vi "1A Interpret NMEA Sentence.vi"(10 "Defilter Wind Data":bool=TRUE, 11 "NMEA Sentence":string) -> ()   [LabVIEW 2011]
doc: "Interprets the NMEA 0813 sentences that we are using from our Airmar PB200 WeatherStation sensor.\nBy Jaime McCandless\nTODO: finish implementing NMEA sentences"
uses:
  2-Think/2 Typedefs/UTM Location.ctl
  2-Think/2 Typedefs/heading.ctl
  2-Think/2 Typedefs/Velocity.ctl
  2-Think/2 Typedefs/apparent wind.ctl
  2-Think/2 Typedefs/pitch and roll.ctl
  2-Think/2 Globals/2 Global.vi
  <vilib>/regexp/Match Regular Expression.xnode
panel:
  out "Meteorological Data":T1
  in  "UTC Time Zone":i32=-5
  in  "Tab Control":T2(tab)
  out "GPS (GGA) Data":T3
  out "GPS (GLL) Data":T4
  out "GPGSA Data":T5
  out "UTC Time":timestamp
  out "Local Time":timestamp
  out "Lattitude (ddmm.mmmm)":dbl format="%_8g"
  out "Lattitude North/South":string
  out "Longitude (ddmm.mmmm)":dbl format="%_8g"
  out "Longitude East/West":string
  out "Speed over ground (knots)":dbl format="%_3g"
  out "Course over ground (degrees)":dbl format="%_4g"
  out "Magnetic Variation (degrees)":dbl format="%_4g"
  out "Variation East/West":string
  out "GPS (RMC) Data":T6 {"Course over ground (degrees)" format="%#.6g"; "Speed over ground (knots)" format="%#.6g"; "Magnetic Variation (degrees)" format="%#.6g"; "Longitude (ddmm.mmmm)" format="%#.6g"; "Lattitude (ddmm.mmmm)" format="%#.6g"}
  out "GPS Data Valid?":bool
  out "Robot UTM Location":T7 {"North" format="%#_10f"; "East" format="%#_8f"}
  out "GPS (VTG) Data":T8
  out "Heading":dbl
  out "Turn (ROT) Data":T9
  out "Wind (MWV) Data":T10
  out "Transducer (XDR) B Data":cluster{"Pitch (deg)":dbl, "Roll (deg)":dbl}
  out "Transducer (XDR) A Data":T11
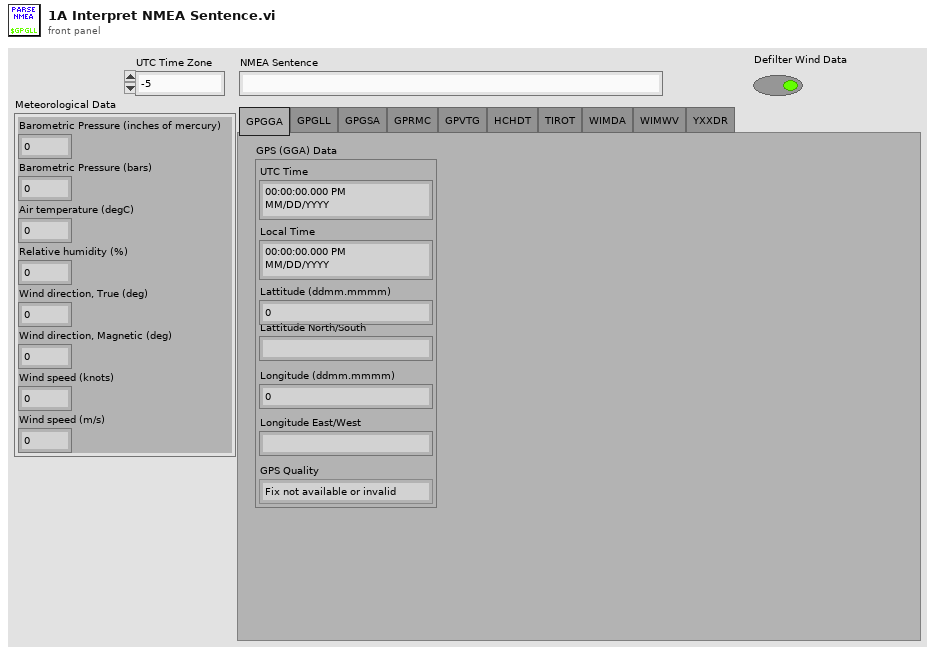
[diagram p1: front panel]
types:
  T1 = cluster{"Barometric Pressure (inches of mercury)":dbl, "Barometric Pressure (bars)":dbl, "Air temperature (degC)":dbl, "Relative humidity (%)":dbl, "Wind direction, True (deg)":dbl, "Wind direction, Magnetic (deg)":dbl, "Wind speed (knots)":dbl, "Wind speed (m/s)":dbl}
  T2 = enum32{"GPGGA", "GPGLL", "GPGSA", "GPRMC", "GPVTG", "HCHDT", "TIROT", "WIMDA", "WIMWV", "YXXDR"}
  T3 = cluster{"UTC Time":timestamp, "Local Time":timestamp, "Lattitude (ddmm.mmmm)":dbl, "Lattitude North/South":string, "Longitude (ddmm.mmmm)":dbl, "Longitude East/West":string, "GPS Quality":enum16{"Fix not available or invalid", "GPS SPS Mode, fix valid", "Differential GPS, SPS Mode, fix valid", "GPS PPS Mode, fix valid", "Real Time Kinematic (RTK)", "Float RTK", "Estimated (dead reckoning) Mode", "Manual Input Mode", "Simulator Mode"}}
  T4 = cluster{"UTC Time":timestamp, "Local Time":timestamp, "Lattitude (ddmm.mmmm)":dbl, "Lattitude North/South":string, "Longitude (ddmm.mmmm)":dbl, "Longitude East/West":string, "GPS Mode":string, "GPS Data Valid?":bool}
  T5 = cluster{"Mode":string, "Fix Strength":i32, "Satellite IDs":i32[], "PDOP":dbl, "HDOP":dbl, "VDOP":dbl}
  T6 = cluster{"UTC Time":timestamp, "Local Time":timestamp, "Lattitude (ddmm.mmmm)":dbl, "Lattitude North/South":string, "Longitude (ddmm.mmmm)":dbl, "Longitude East/West":string, "Magnetic Variation (degrees)":dbl, "Variation East/West":string, "Speed over ground (knots)":dbl, "Course over ground (degrees)":dbl}
  T7 = typedef "UTM Location.ctl" = cluster{"UTM Zone":dbl, "Hemisphere":enum16{"North", "South"}, "East":dbl, "North":dbl}
  T8 = cluster{"Course Over Ground (True)":dbl, "Course Over Ground (Magnetic)":dbl, "Speed Over Ground (Knots)":dbl, "Speed Over Ground (km/hr)":dbl, "GPS Mode":string}
  T9 = cluster{"Rate of Turn (deg/min)":dbl, "Turn Rotation Data Valid?":bool}
  T10 = cluster{"Angle relative to boat (deg)":dbl, "Wind Data Valid?":bool, "Wind speed (knots)":dbl, "True (T) or Relative (R)":string}
  T11 = cluster{"Calc. Relative Wind Chill (degC)":dbl, "Calc. Theoretical Wind Chill (degC)":dbl, "Calc. Heat Index (degC)":dbl, "Meas. Barometric Pressure (bars)":dbl}
  T12 = cluster{"second":i32, "minute":i32, "hour":i32, "day of month":i32, "month":i32, "year":i32, "day of week":i32, "day of year":i32, "is DST":i32}
  T13 = typedef "heading.ctl" = dbl
  T14 = typedef "Velocity.ctl" = cluster{"East":dbl, "North":dbl}
  T15 = typedef "apparent wind.ctl" = cluster{"Toward Fore":dbl, "Toward Starboard":dbl}
  T16 = typedef "pitch and roll.ctl" = cluster{"Pitch":dbl, "Roll":dbl}
  T17 = typedef "generalized sensor status.ctl" = cluster{"Sensor Connected":T18, "Sensor Initialized":T18, "Sensor OK":T18, "Latest Error String":string, "GPS Lock":T18}
  T18 = typedef "indicator LED.ctl" = bool
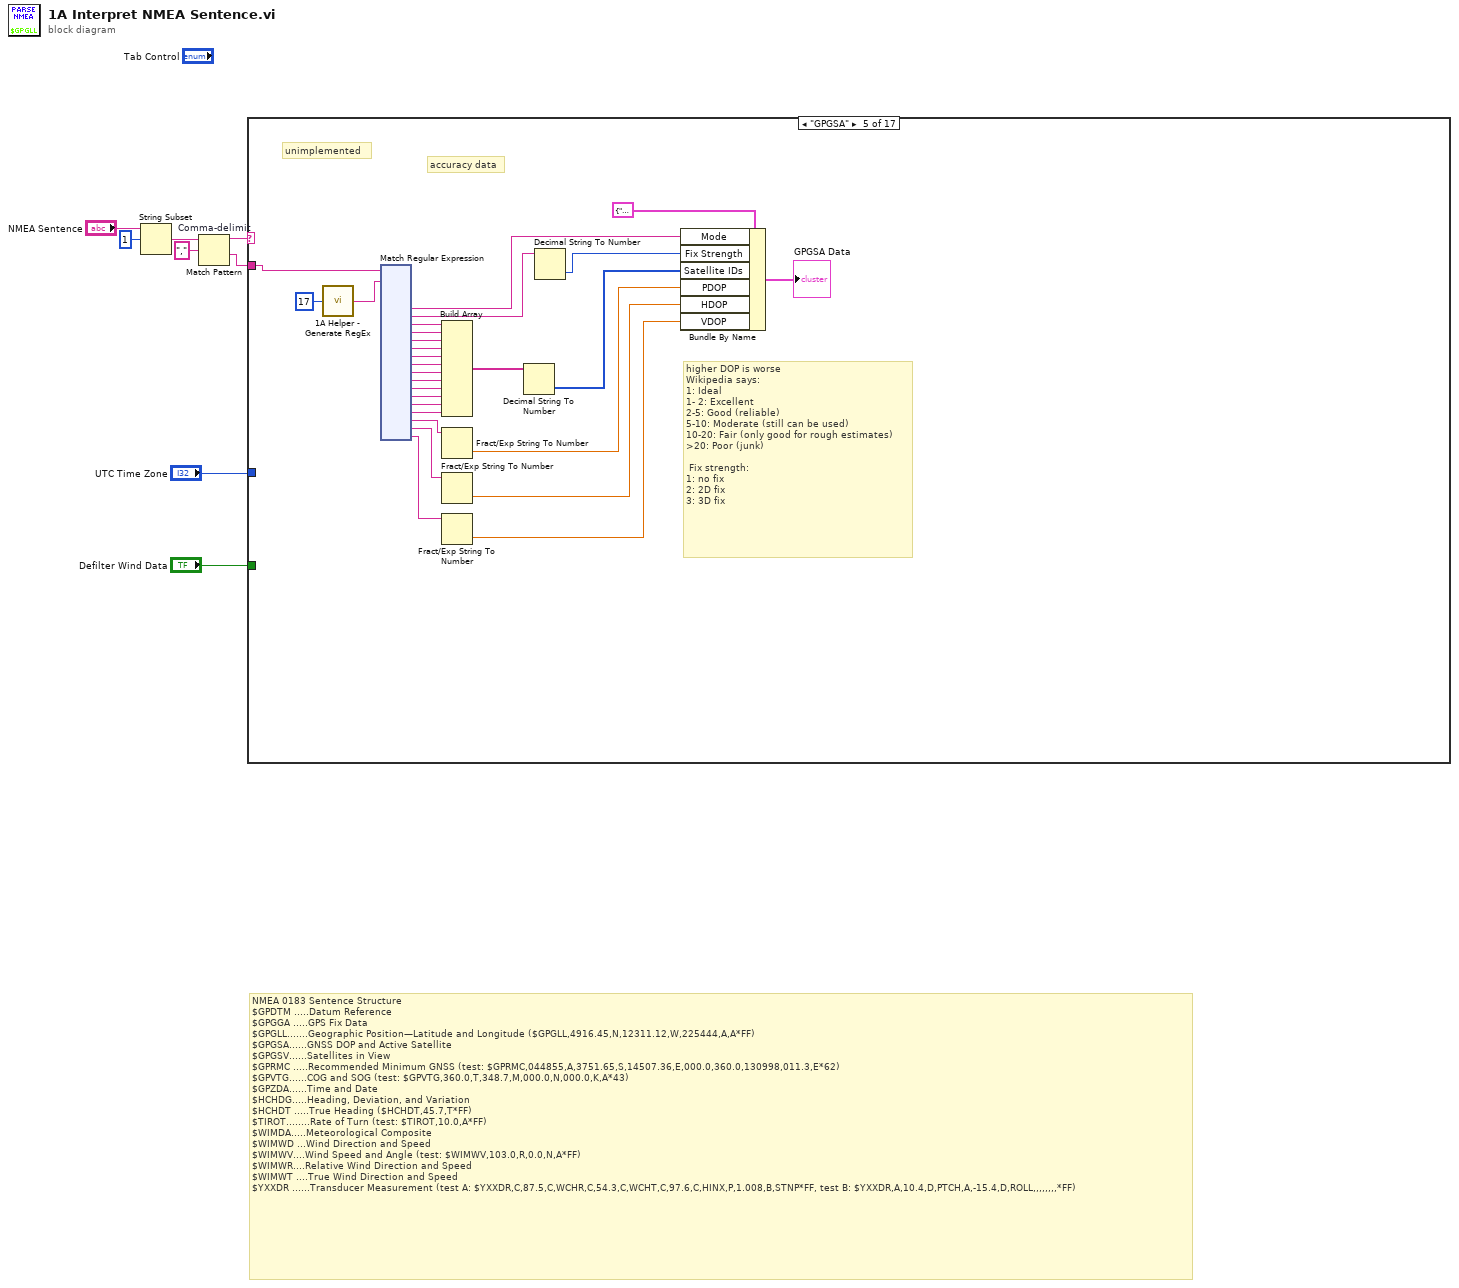
[diagram p0: block diagram]
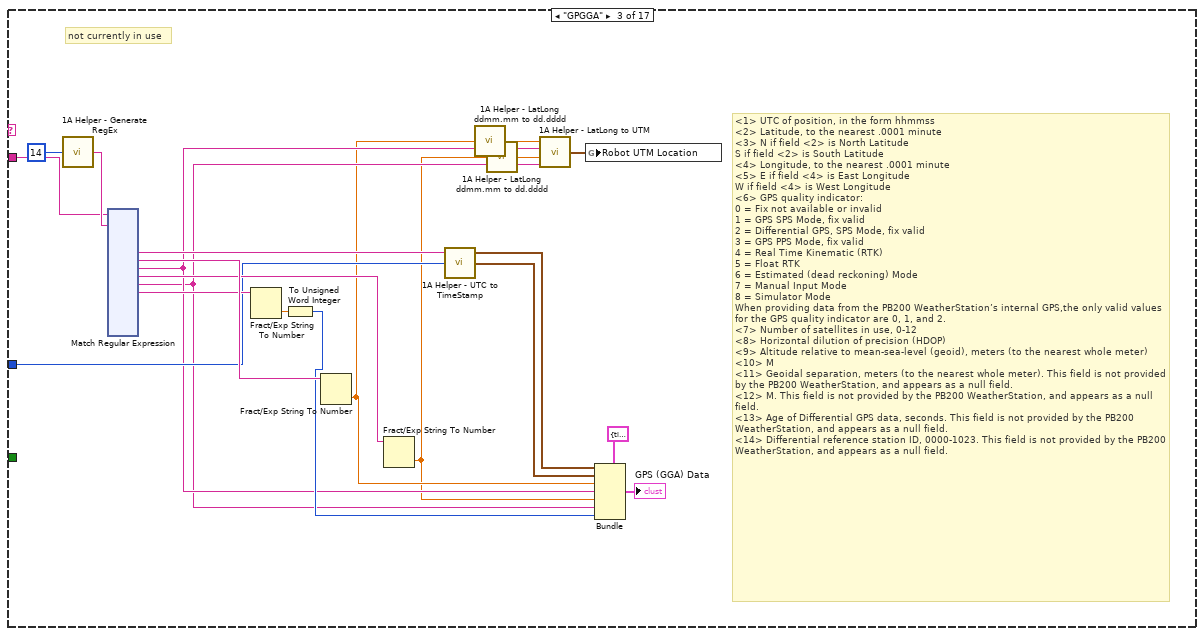
[diagram p4: hidden frame]
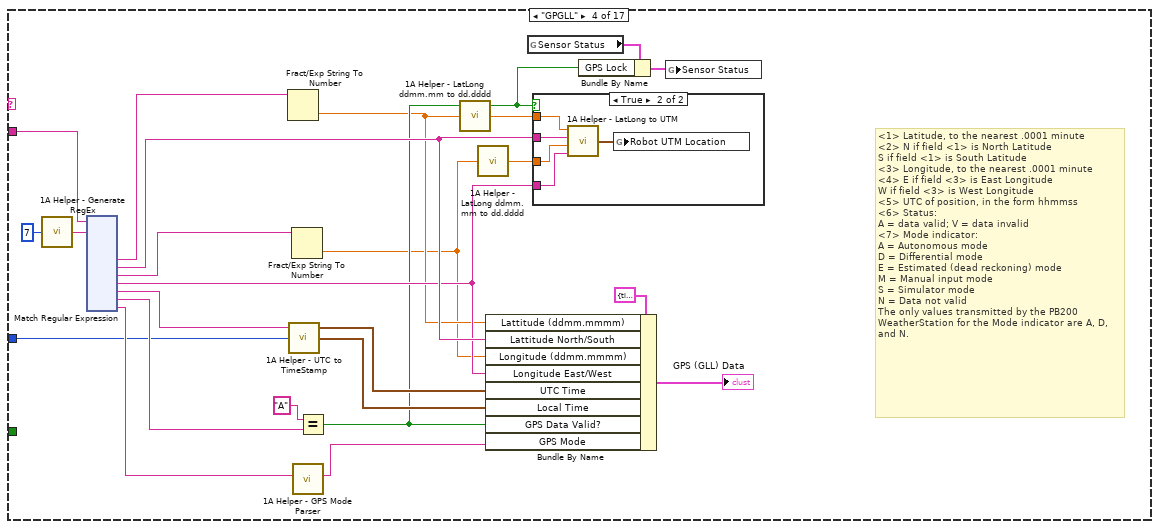
[diagram p5: hidden frame]
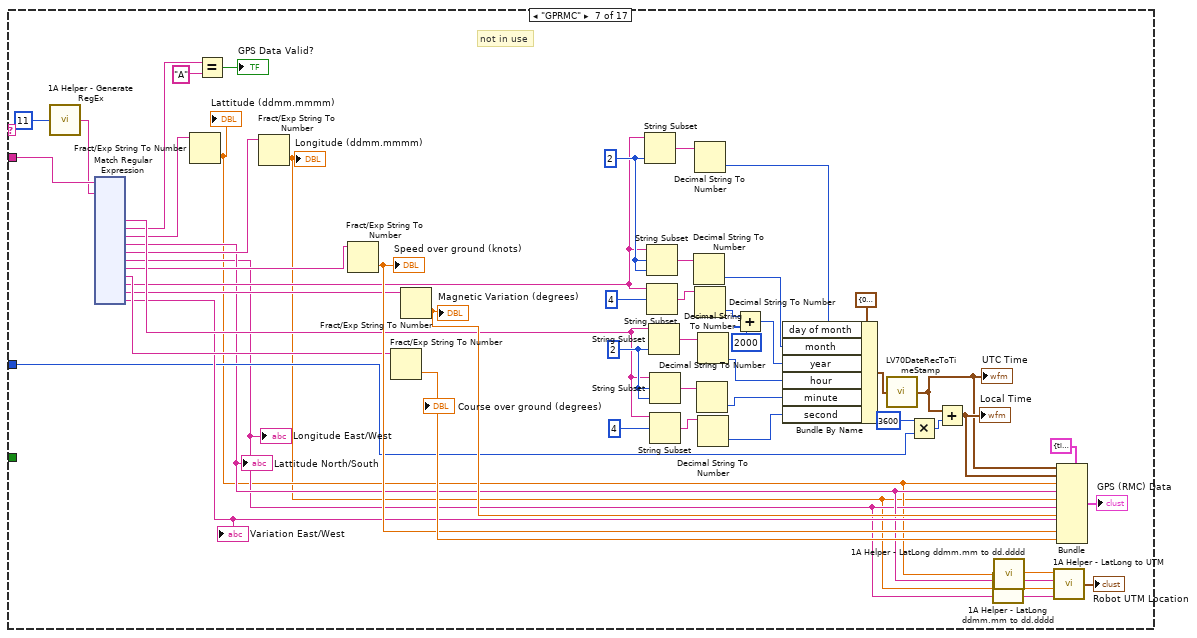
[diagram p8: hidden frame]
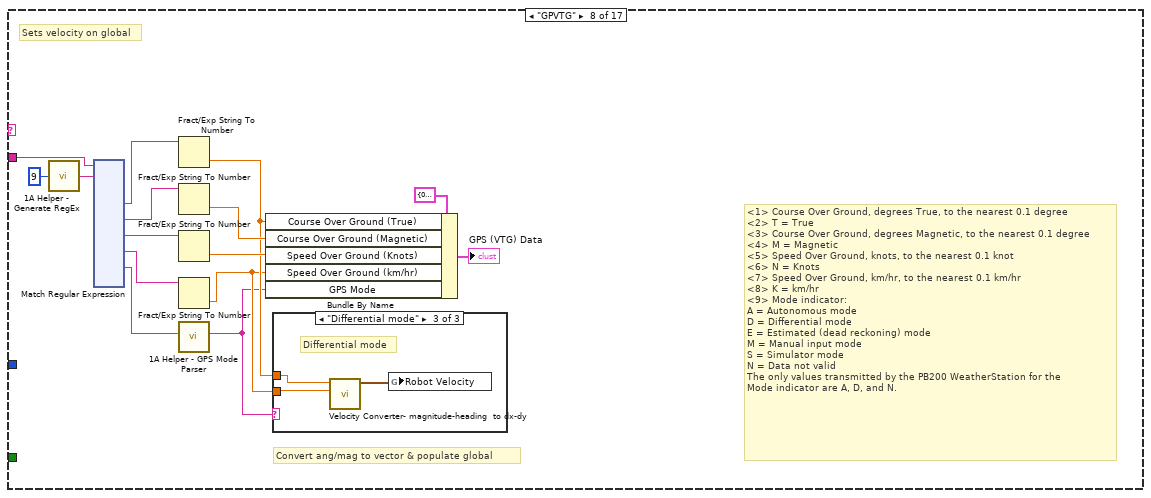
[diagram p9: hidden frame]
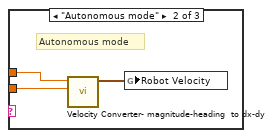
[diagram p11: hidden frame]
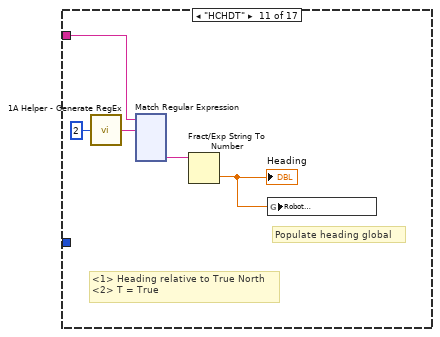
[diagram p14: hidden frame]
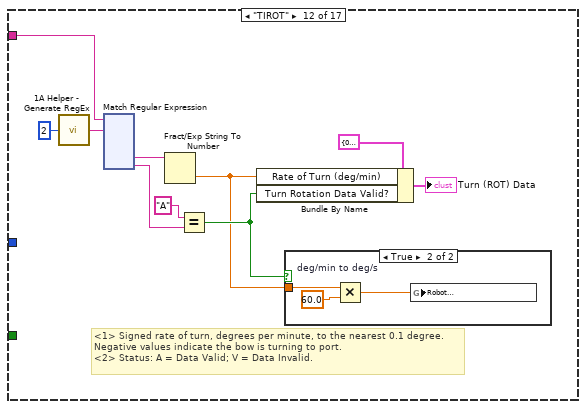
[diagram p15: hidden frame]
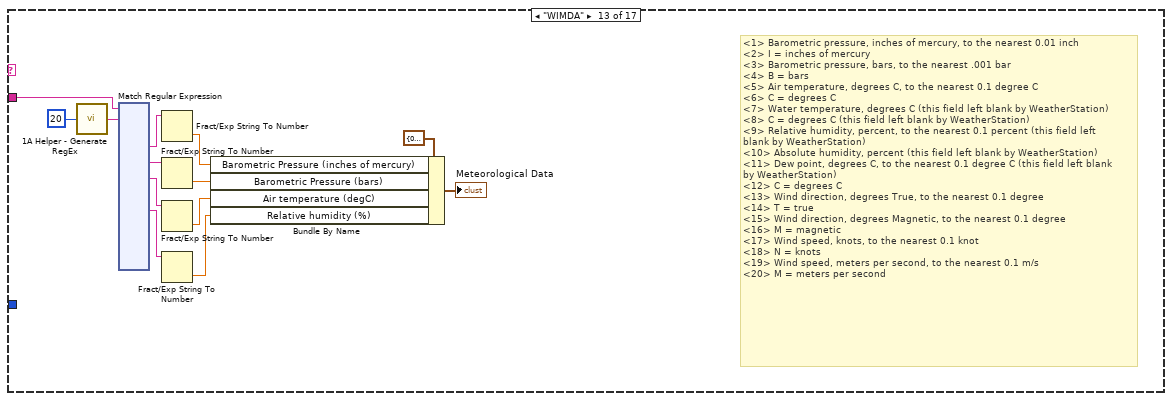
[diagram p17: hidden frame]
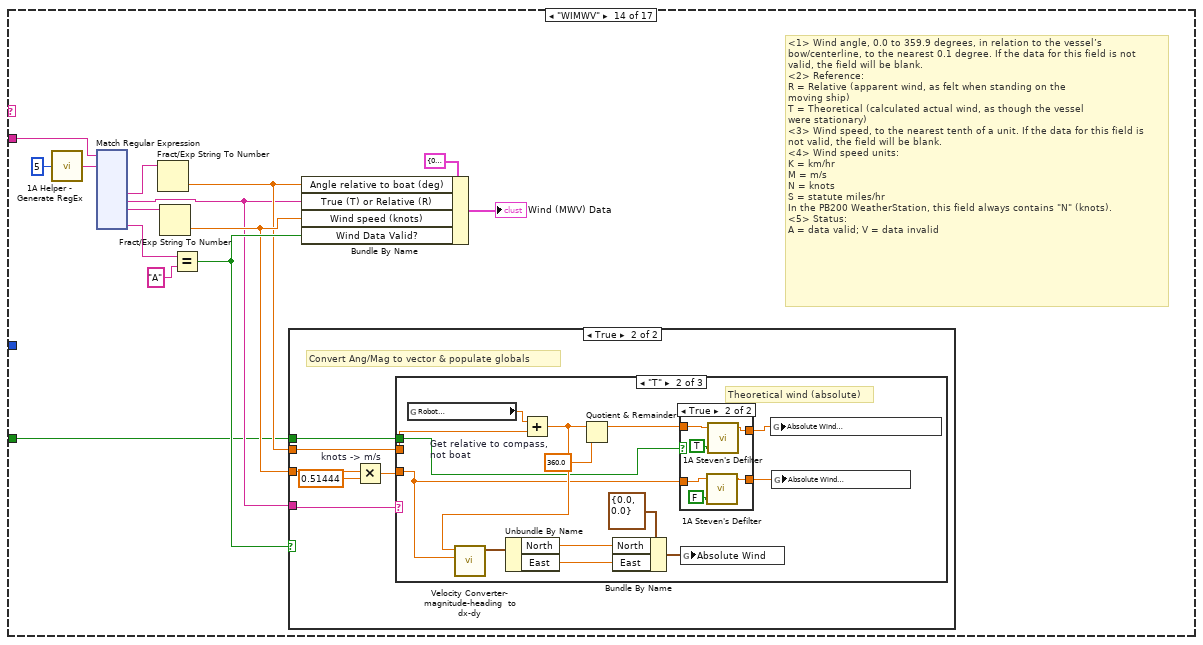
[diagram p18: hidden frame]
diagram:
  # "NMEA 0183 Sentence Structure\n$GPDTM .....Datum Reference\n$GPGGA .....GPS Fix Data\n$GPGLL.......Geographic Position—Latitude and Longitude ($GPGLL,4916.45,N,12311.12,W,225444,A,A*FF)\n$GPGSA......GNSS DOP and Active Satellite\n$GPGSV......Satellites in View\n$GPRMC .....Recommended Minimum GNSS (test: $GPRMC,044855,A,3751.65,S,14507.36,E,000.0,360.0,130998,011.3,E*62)\n$GPVTG......COG and SOG (test: $GPVTG,360.0,T,348.7,M,000.0,N,000.0,K,A*43)\n$GPZDA......Time and Date\n$HCHDG.....Heading, Deviation, and Variation\n$HCHDT .....True Heading ($HCHDT,45.7,T*FF)\n$TIROT........Rate of Turn (test: $TIROT,10.0,A*FF)\n$WIMDA.....Meteorological Composite\n$WIMWD ...Wind Direction and Speed\n$WIMWV....Wind Speed and Angle (test: $WIMWV,103.0,R,0.0,N,A*FF)\n$WIMWR....Relative Wind Direction and Speed\n$WIMWT ....True Wind Direction and Speed\n$YXXDR ......Transducer Measurement (test A: $YXXDR,C,87.5,C,WCHR,C,54.3,C,WCHT,C,97.6,C,HINX,P,1.008,B,STNP*FF, test B: $YXXDR,A,10.4,D,PTCH,A,-15.4,D,ROLL,,,,,,,,*FF)"
  n1 = String Subset(string="NMEA Sentence", offset (0)=1) -> (substring=w5:string)  [unwired: 1 in]
  n2 = Match Pattern "Comma-delimit"(string=w5, regular expression=",") -> (before substring=w6:string, after substring=w7:string)  [unwired: 1 in, 2 out]
  n3 = case shown="\"GPGSA\"" w6 {
    tunnel: w7 -> [_ _ w27 w171 w328 _ w477 w644 _ _ w778 w900 w1031 w1171 _ _ w1339]
    tunnel: "UTC Time Zone" -> [_ _ w16 w163 _ _ w465 _ _ _ _ _ _ _ _ _ _]
    tunnel: "Defilter Wind Data" -> [_ _ _ _ _ _ _ _ _ _ _ _ _ w1162 _ _ _]
    frame "", Default {
    }
    frame "GPDTM" {
      # "unimplemented"
    }
    frame "GPGGA" {
      # "not currently in use"
      # "<1> UTC of position, in the form hhmmss\n<2> Latitude, to the nearest .0001 minute\n<3> N if field <2> is North Latitude\nS if field <2> is South Latitude\n<4> Longitude, to the nearest .0001 minute\n<5> E if field <4> is East Longitude\nW if field <4> is West Longitude\n<6> GPS quality indicator:\n0 = Fix not available or invalid\n1 = GPS SPS Mode, fix valid\n2 = Differential GPS, SPS Mode, fix valid\n3 = GPS PPS Mode, fix valid\n4 = Real Time Kinematic (RTK)\n5 = Float RTK\n6 = Estimated (dead reckoning) Mode\n7 = Manual Input Mode\n8 = Simulator Mode\nWhen providing data from the PB200 WeatherStation’s internal GPS,the only valid values for the GPS quality indicator are 0, 1, and 2.\n<7> Number of satellites in use, 0-12\n<8> Horizontal dilution of precision (HDOP)\n<9> Altitude relative to mean-sea-level (geoid), meters (to the nearest whole meter)\n<10> M\n<11> Geoidal separation, meters (to the nearest whole meter). This field is not provided by the PB200 WeatherStation, and appears as a null field.\n<12> M. This field is not provided by the PB200 WeatherStation, and appears as a null field.\n<13> Age of Differential GPS data, seconds. This field is not provided by the PB200 WeatherStation, and appears as a null field.\n<14> Differential reference station ID, 0000-1023. This field is not provided by the PB200 WeatherStation, and appears as a null field."
      n4 = call "1A Helper - Generate RegEx.vi"("# Datums"=14) -> ("RegEx"=w28:string)
      n5 = xnode "Match Regular Expression"("input string"=w27, "regular expression"=w28) -> ("submatch 1"=w19:string, "submatch 2"=w25:string, "submatch 3"=w14:string, "submatch 4"=w24:string, "submatch 5"=w13:string, "submatch 6"=w23:string)  [unwired: 4 in, 10 out]
      n6 = Fract/Exp String To Number(string=w23) -> (number=w22:dbl)  [unwired: 3 in, 1 out]
      n7 = To Unsigned Word Integer(number=w22) -> (unsigned 16bit integer=w21:u16)
      n8 = Fract/Exp String To Number(string=w25) -> (number=w11:dbl)  [unwired: 3 in, 1 out]
      n9 = Fract/Exp String To Number(string=w24) -> (number=w9:dbl)  [unwired: 3 in, 1 out]
      n10 = call "1A Helper - UTC to TimeStamp.vi"("UTC Time Zone in"=w16, "UTC (hhmmss)"=w19) -> ("Local Time"=w17:timestamp, "UTC Time"=w18:timestamp)  [unwired: 2 in]
      n11 = call "1A Helper - LatLong ddmm.mm to dd.dddd.vi"("Lattitude/Longitude in ddmm.mmmm"=w11) -> ("Latitude/Longitude in dd.dddddd"=w12:dbl)
      n12 = call "1A Helper - LatLong ddmm.mm to dd.dddd.vi"("Lattitude/Longitude in ddmm.mmmm"=w9) -> ("Latitude/Longitude in dd.dddddd"=w10:dbl)
      n13 = call "1A Helper - LatLong to UTM.vi"("East/West"=w13, "Longitude"=w10, "North/South"=w14, "Latitude"=w12) -> ("Robot UTM Location"=w15:T7)
      n14 = global write "2 Global.vi" "Robot UTM Location"(w15) -> ()
      n15 = Bundle(cluster=T3 {"UTC Time"=timestamp(0 s since 1904-01-01), "Local Time"=timestamp(0 s since 1904-01-01), "Lattitude (ddmm.mmmm)"=0.0, "Lattitude North/South"="", "Longitude (ddmm.mmmm)"=0.0, "Longitude East/West"="", "GPS Quality"=enum."GPS SPS Mode, fix valid"} ("Cluster"), "UTC Time"=w18, "Local Time"=w17, "Lattitude (ddmm.mmmm)"=w11, "Lattitude North/South"=w14, "Longitude (ddmm.mmmm)"=w9, "Longitude East/West"=w13, "GPS Quality"=w21) -> (→"GPS (GGA) Data":T3)
    }
    frame "GPGLL" {
      # "<1> Latitude, to the nearest .0001 minute\n<2> N if field <1> is North Latitude\nS if field <1> is South Latitude\n<3> Longitude, to the nearest .0001 minute\n<4> E if field <3> is East Longitude\nW if field <3> is West Longitude\n<5> UTC of position, in the form hhmmss\n<6> Status:\nA = data valid; V = data invalid\n<7> Mode indicator:\nA = Autonomous mode\nD = Differential mode\nE = Estimated (dead reckoning) mode\nM = Manual input mode\nS = Simulator mode\nN = Data not valid\nThe only values transmitted by the PB200 WeatherStation for the Mode indicator are A, D, and N."
      n16 = call "1A Helper - Generate RegEx.vi"("# Datums"=7) -> ("RegEx"=w175:string)
      n17 = xnode "Match Regular Expression"("input string"=w171, "regular expression"=w175) -> ("submatch 1"=w174:string, "submatch 2"=w161:string, "submatch 3"=w173:string, "submatch 4"=w160:string, "submatch 5"=w170:string, "submatch 6"=w166:string, "submatch 7"=w172:string)  [unwired: 4 in, 5 out]
      n18 = Fract/Exp String To Number(string=w174) -> (number=w156:dbl)  [unwired: 3 in, 1 out]
      n19 = call "1A Helper - UTC to TimeStamp.vi"("UTC Time Zone in"=w163, "UTC (hhmmss)"=w170) -> ("Local Time"=w165:timestamp, "UTC Time"=w164:timestamp)  [unwired: 2 in]
      n20 = Fract/Exp String To Number(string=w173) -> (number=w154:dbl)  [unwired: 3 in, 1 out]
      n21 = call "1A Helper - GPS Mode Parser.vi"("GPS Mode (Char)"=w172) -> ("GPS Mode (Description)"=w168:string)  [unwired: 6 in]
      n22 = Equal?(x="A" ("y"), y=w166) -> (x = y?=w157:bool)
      n23 = call "1A Helper - LatLong ddmm.mm to dd.dddd.vi"("Lattitude/Longitude in ddmm.mmmm"=w156) -> ("Latitude/Longitude in dd.dddddd"=w155:dbl)
      n24 = call "1A Helper - LatLong ddmm.mm to dd.dddd.vi"("Lattitude/Longitude in ddmm.mmmm"=w154) -> ("Latitude/Longitude in dd.dddddd"=w153:dbl)
      n25 = Bundle By Name(cluster=T4 {"UTC Time"=timestamp(0 s since 1904-01-01), "Local Time"=timestamp(0 s since 1904-01-01), "Lattitude (ddmm.mmmm)"=0.0, "Lattitude North/South"="", "Longitude (ddmm.mmmm)"=0.0, "Longitude East/West"="", "GPS Mode"="", "GPS Data Valid?"=FALSE} ("Cluster"), "Lattitude (ddmm.mmmm)"=w156, "Lattitude North/South"=w161, "Longitude (ddmm.mmmm)"=w154, "Longitude East/West"=w160, "UTC Time"=w164, "Local Time"=w165, "GPS Data Valid?"=w157, "GPS Mode"=w168) -> (→"GPS (GLL) Data":T4)
      n26 = global read "2 Global.vi" "Sensor Status"() -> (w158:T17)
      n27 = case shown="True" w157 {
        tunnel: w155 -> [_ w181]
        tunnel: w161 -> [_ w180]
        tunnel: w153 -> [_ w179]
        tunnel: w160 -> [_ w178]
        frame False {
        }
        frame True {
          n28 = call "1A Helper - LatLong to UTM.vi"("East/West"=w178, "Longitude"=w179, "North/South"=w180, "Latitude"=w181) -> ("Robot UTM Location"=w177:T7)
          n29 = global write "2 Global.vi" "Robot UTM Location"(w177) -> ()
        }
      }
      n30 = Bundle By Name(cluster=w158, "GPS Lock"=w157) -> (w159:T17)
      n31 = global write "2 Global.vi" "Sensor Status"(w159) -> ()
    }
    frame "GPGSA" {
      # "higher DOP is worse\nWikipedia says:\n1: Ideal\n1- 2: Excellent\n2-5: Good (reliable)\n5-10: Moderate (still can be used)\n10-20: Fair (only good for rough estimates)\n>20: Poor (junk)\n\n Fix strength: \n1: no fix\n2: 2D fix\n3: 3D fix"
      # "accuracy data"
      # "unimplemented"
      n32 = call "1A Helper - Generate RegEx.vi"("# Datums"=17) -> ("RegEx"=w327:string)
      n33 = xnode "Match Regular Expression"("input string"=w328, "regular expression"=w327) -> ("submatch 1"=w324:string, "submatch 2"=w323:string, "submatch 3"=w321:string, "submatch 4"=w320:string, "submatch 5"=w319:string, "submatch 6"=w318:string, "submatch 7"=w317:string, "submatch 8"=w316:string, "submatch 9"=w315:string, "submatch 10"=w314:string, "submatch 11"=w313:string, "submatch 12"=w312:string, "submatch 13"=w311:string, "submatch 14"=w310:string, "submatch 15"=w307:string, "submatch 16"=w305:string, "submatch 17"=w303:string)  [unwired: 4 in, 5 out]
      n34 = Build Array(w321, w320, w319, w318, w317, w316, w315, w314, w313, w312, w311, w310) -> (w309:string[])
      n35 = Fract/Exp String To Number(string=w307) -> (number=w306:dbl)  [unwired: 3 in, 1 out]
      n36 = Fract/Exp String To Number(string=w305) -> (number=w304:dbl)  [unwired: 3 in, 1 out]
      n37 = Fract/Exp String To Number(string=w303) -> (number=w302:dbl)  [unwired: 3 in, 1 out]
      n38 = Decimal String To Number(string=w309) -> (number=w308:i32[])  [unwired: 2 in, 1 out]
      n39 = Decimal String To Number(string=w323) -> (number=w322:i32)  [unwired: 2 in, 1 out]
      n40 = Bundle By Name(cluster=T5 {"Mode"="", "Fix Strength"=0, "Satellite IDs"=[], "PDOP"=0.0, "HDOP"=0.0, "VDOP"=0.0} ("GPGSA Data"), "Mode"=w324, "Fix Strength"=w322, "Satellite IDs"=w308, "PDOP"=w306, "HDOP"=w304, "VDOP"=w302) -> (→"GPGSA Data":T5)
    }
    frame "GPGSV" {
      # "unimplemented"
    }
    frame "GPRMC" {
      w495 = 2 ("length (rest)")
      w485 = 2 ("length (rest)")
      # "not in use"
      n41 = call "1A Helper - Generate RegEx.vi"("# Datums"=11) -> ("RegEx"=w467:string)
      n42 = xnode "Match Regular Expression"("input string"=w477, "regular expression"=w467) -> ("submatch 1"=w476:string, "submatch 2"=w475:string, "submatch 3"=w474:string, "submatch 4"=w464:string, "submatch 5"=w473:string, "submatch 6"=w463:string, "submatch 7"=w472:string, "submatch 8"=w471:string, "submatch 9"=w470:string, "submatch 10"=w469:string, "submatch 11"=w468:string)  [unwired: 4 in, 5 out]
      "Lattitude North/South" <- w464
      "Longitude East/West" <- w463
      "Variation East/West" <- w468
      n43 = Fract/Exp String To Number(string=w474) -> (number=w460:dbl)  [unwired: 3 in, 1 out]
      "Lattitude (ddmm.mmmm)" <- w460
      n44 = Equal?(x=w475, y="A") -> (x = y?=→"GPS Data Valid?":bool)
      n45 = Fract/Exp String To Number(string=w473) -> (number=w458:dbl)  [unwired: 3 in, 1 out]
      "Longitude (ddmm.mmmm)" <- w458
      n46 = Fract/Exp String To Number(string=w472) -> (number=w505:dbl)  [unwired: 3 in, 1 out]
      "Speed over ground (knots)" <- w505
      n47 = Fract/Exp String To Number(string=w471) -> (number=w506:dbl)  [unwired: 3 in, 1 out]
      "Course over ground (degrees)" <- w506
      n48 = Fract/Exp String To Number(string=w469) -> (number=w504:dbl)  [unwired: 3 in, 1 out]
      "Magnetic Variation (degrees)" <- w504
      n49 = String Subset(string=w470, length (rest)=w495) -> (substring=w496:string)  [unwired: 1 in]
      n50 = String Subset(string=w470, offset (0)=w495, length (rest)=w495) -> (substring=w494:string)
      n51 = String Subset(string=w470, offset (0)=4) -> (substring=w492:string)  [unwired: 1 in]
      n52 = String Subset(string=w476, length (rest)=w485) -> (substring=w481:string)  [unwired: 1 in]
      n53 = String Subset(string=w476, offset (0)=w485, length (rest)=w485) -> (substring=w487:string)
      n54 = String Subset(string=w476, offset (0)=4) -> (substring=w489:string)  [unwired: 1 in]
      n55 = Decimal String To Number(string=w494) -> (number=w498:i32)  [unwired: 2 in, 1 out]
      n56 = Decimal String To Number(string=w496) -> (number=w497:i32)  [unwired: 2 in, 1 out]
      n57 = Decimal String To Number(string=w492) -> (number=w499:i32)  [unwired: 2 in, 1 out]
      n58 = Decimal String To Number(string=w487) -> (number=w486:i32)  [unwired: 2 in, 1 out]
      n59 = Decimal String To Number(string=w481) -> (number=w484:i32)  [unwired: 2 in, 1 out]
      n60 = Decimal String To Number(string=w489) -> (number=w490:i32)  [unwired: 2 in, 1 out]
      n61 = Add(x=w499, y=2000) -> (x+y=w501:i32)
      n62 = Bundle By Name(cluster=T12 {"second"=0, "minute"=0, "hour"=0, "day of month"=0, "month"=0, "year"=0, "day of week"=0, "day of year"=0, "is DST"=0} ("date time rec"), "day of month"=w497, "month"=w498, "year"=w501, "hour"=w484, "minute"=w486, "second"=w490) -> (w482:T12)
      n63 = call <vilib>:"LV70DateRecToTimeStamp.vi"("date time rec"=w482) -> ("Time Stamp"=w502:timestamp)
      "UTC Time" <- w502
      n64 = Multiply(x=3600 ("number"), y=w465) -> (x*y=w466:i32)
      n65 = Add(x=w502, y=w466) -> (x+y=w503:timestamp)
      "Local Time" <- w503
      n66 = call "1A Helper - LatLong ddmm.mm to dd.dddd.vi"("Lattitude/Longitude in ddmm.mmmm"=w458) -> ("Latitude/Longitude in dd.dddddd"=w459:dbl)
      n67 = call "1A Helper - LatLong ddmm.mm to dd.dddd.vi"("Lattitude/Longitude in ddmm.mmmm"=w460) -> ("Latitude/Longitude in dd.dddddd"=w461:dbl)
      n68 = call "1A Helper - LatLong to UTM.vi"("East/West"=w463, "Longitude"=w459, "North/South"=w464, "Latitude"=w461) -> ("Robot UTM Location"=→"Robot UTM Location":T7)
      n69 = Bundle(cluster=T6 {"UTC Time"=timestamp(0 s since 1904-01-01), "Local Time"=timestamp(0 s since 1904-01-01), "Lattitude (ddmm.mmmm)"=0.0, "Lattitude North/South"="", "Longitude (ddmm.mmmm)"=0.0, "Longitude East/West"="", "Magnetic Variation (degrees)"=0.0, "Variation East/West"="", "Speed over ground (knots)"=0.0, "Course over ground (degrees)"=0.0} ("Cluster"), "UTC Time"=w502, "Local Time"=w503, "Lattitude (ddmm.mmmm)"=w460, "Lattitude North/South"=w464, "Longitude (ddmm.mmmm)"=w458, "Longitude East/West"=w463, "Magnetic Variation (degrees)"=w504, "Variation East/West"=w468, "Speed over ground (knots)"=w505, "Course over ground (degrees)"=w506) -> (→"GPS (RMC) Data":T6)
    }
    frame "GPVTG" {
      # "Convert ang/mag to vector & populate global"
      # "Sets velocity on global"
      # "<1> Course Over Ground, degrees True, to the nearest 0.1 degree\n<2> T = True\n<3> Course Over Ground, degrees Magnetic, to the nearest 0.1 degree\n<4> M = Magnetic\n<5> Speed Over Ground, knots, to the nearest 0.1 knot\n<6> N = Knots\n<7> Speed Over Ground, km/hr, to the nearest 0.1 km/hr\n<8> K = km/hr\n<9> Mode indicator:\nA = Autonomous mode\nD = Differential mode\nE = Estimated (dead reckoning) mode\nM = Manual input mode\nS = Simulator mode\nN = Data not valid\nThe only values transmitted by the PB200 WeatherStation for the\nMode indicator are A, D, and N."
      n70 = call "1A Helper - Generate RegEx.vi"("# Datums"=9) -> ("RegEx"=w645:string)
      n71 = xnode "Match Regular Expression"("input string"=w644, "regular expression"=w645) -> ("submatch 1"=w641:string, "submatch 3"=w640:string, "submatch 5"=w638:string, "submatch 7"=w636:string, "submatch 9"=w635:string)  [unwired: 4 in, 11 out]
      n72 = Fract/Exp String To Number(string=w641) -> (number=w634:dbl)  [unwired: 3 in, 1 out]
      n73 = Fract/Exp String To Number(string=w640) -> (number=w639:dbl)  [unwired: 3 in, 1 out]
      n74 = Fract/Exp String To Number(string=w638) -> (number=w637:dbl)  [unwired: 3 in, 1 out]
      n75 = Fract/Exp String To Number(string=w636) -> (number=w633:dbl)  [unwired: 3 in, 1 out]
      n76 = call "1A Helper - GPS Mode Parser.vi"("GPS Mode (Char)"=w635) -> ("GPS Mode (Description)"=w632:string)  [unwired: 6 in]
      n77 = Bundle By Name(cluster=T8 {"Course Over Ground (True)"=0.0, "Course Over Ground (Magnetic)"=0.0, "Speed Over Ground (Knots)"=0.0, "Speed Over Ground (km/hr)"=0.0, "GPS Mode"=""} ("GPS (VTG) Data 2"), "Course Over Ground (True)"=w634, "Course Over Ground (Magnetic)"=w639, "Speed Over Ground (Knots)"=w637, "Speed Over Ground (km/hr)"=w633, "GPS Mode"=w632) -> (→"GPS (VTG) Data":T8)
      n78 = case shown="\"Differential mode\"" w632 {
        tunnel: w634 -> [_ w649 w652]
        tunnel: w633 -> [_ w648 w651]
        frame "Data not valid", Default {
          # "Data not valid"
        }
        frame "Autonomous mode" {
          # "Autonomous mode"
          n79 = call "Velocity Converter- magnitude-heading  to dx-dy.vi"("Magnitude"=w648, "Heading"=w649) -> ("Vector Out"=w647:T14)  [unwired: 9 in]
          n80 = global write "2 Global.vi" "Robot Velocity"(w647) -> ()
        }
        frame "Differential mode" {
          # "Differential mode"
          n81 = call "Velocity Converter- magnitude-heading  to dx-dy.vi"("Magnitude"=w651, "Heading"=w652) -> ("Vector Out"=w650:T14)  [unwired: 9 in]
          n82 = global write "2 Global.vi" "Robot Velocity"(w650) -> ()
        }
      }
    }
    frame "GPZDA" {
      # "<1> UTC time of day, in the form hhmmss\n<2> UTC day, 01 to 31\n<3> UTC month, 01 to 12\n<4> UTC year (four digits, e.g. 2006)\n<5> Local time zone hours, 00 to +/-13 hrs\n<6> Local time zone minutes, 00 to +59"
    }
    frame "HCHDG " {
      # "<1> Magnetic sensor heading, degrees, to the nearest 0.1 degree.\n<2> Magnetic deviation, degrees east or west, to the nearest 0.1 degree.\n<3> E if field <2> is degrees East\nW if field <2> is degrees West\n<4> Magnetic variation, degrees east or west, to the nearest 0.1 degree.\n<5> E if field <4> is degrees East\nW if field <4> is degrees West"
    }
    frame "HCHDT" {
      # "Populate heading global"
      # "<1> Heading relative to True North\n<2> T = True"
      n83 = call "1A Helper - Generate RegEx.vi"("# Datums"=2) -> ("RegEx"=w779:string)
      n84 = xnode "Match Regular Expression"("input string"=w778, "regular expression"=w779) -> ("submatch 1"=w777:string)  [unwired: 4 in, 5 out]
      n85 = Fract/Exp String To Number(string=w777) -> (number=w776:dbl)  [unwired: 3 in, 1 out]
      "Heading" <- w776
      n86 = global write "2 Global.vi" "Robot\nHeading"(w776) -> ()
    }
    frame "TIROT" {
      # "<1> Signed rate of turn, degrees per minute, to the nearest 0.1 degree.\nNegative values indicate the bow is turning to port.\n<2> Status: A = Data Valid; V = Data Invalid."
      n87 = call "1A Helper - Generate RegEx.vi"("# Datums"=2) -> ("RegEx"=w902:string)
      n88 = xnode "Match Regular Expression"("input string"=w900, "regular expression"=w902) -> ("submatch 1"=w901:string, "submatch 2"=w896:string)  [unwired: 4 in, 5 out]
      n89 = Fract/Exp String To Number(string=w901) -> (number=w894:dbl)  [unwired: 3 in, 1 out]
      n90 = Equal?(x="A" ("y"), y=w896) -> (x = y?=w895:bool)
      n91 = Bundle By Name(cluster=T9 {"Rate of Turn (deg/min)"=0.0, "Turn Rotation Data Valid?"=TRUE} ("Turn (ROT) Data 2"), "Rate of Turn (deg/min)"=w894, "Turn Rotation Data Valid?"=w895) -> (→"Turn (ROT) Data":T9)
      n92 = case shown="True" w895 {
        tunnel: w894 -> [_ w905]
        frame False {
        }
        frame True {
          n93 = Multiply "deg/min to deg/s"(x=w905, y=60.0) -> (x*y=w906:dbl)
          n94 = global write "2 Global.vi" "Robot\nRate of Turn"(w906) -> ()
        }
      }
    }
    frame "WIMDA" {
      # "<1> Barometric pressure, inches of mercury, to the nearest 0.01 inch\n<2> I = inches of mercury\n<3> Barometric pressure, bars, to the nearest .001 bar\n<4> B = bars\n<5> Air temperature, degrees C, to the nearest 0.1 degree C\n<6> C = degrees C\n<7> Water temperature, degrees C (this field left blank by WeatherStation)\n<8> C = degrees C (this field left blank by WeatherStation)\n<9> Relative humidity, percent, to the nearest 0.1 percent (this field left\nblank by WeatherStation)\n<10> Absolute humidity, percent (this field left blank by WeatherStation)\n<11> Dew point, degrees C, to the nearest 0.1 degree C (this field left blank\nby WeatherStation)\n<12> C = degrees C\n<13> Wind direction, degrees True, to the nearest 0.1 degree\n<14> T = true\n<15> Wind direction, degrees Magnetic, to the nearest 0.1 degree\n<16> M = magnetic\n<17> Wind speed, knots, to the nearest 0.1 knot\n<18> N = knots\n<19> Wind speed, meters per second, to the nearest 0.1 m/s\n<20> M = meters per second"
      n95 = call "1A Helper - Generate RegEx.vi"("# Datums"=20) -> ("RegEx"=w1032:string)
      n96 = xnode "Match Regular Expression"("input string"=w1031, "regular expression"=w1032) -> ("submatch 1"=w1025:string, "submatch 3"=w1024:string, "submatch 5"=w1023:string, "submatch 9"=w1022:string)  [unwired: 4 in, 17 out]
      n97 = Fract/Exp String To Number(string=w1025) -> (number=w1029:dbl)  [unwired: 3 in, 1 out]
      n98 = Fract/Exp String To Number(string=w1024) -> (number=w1028:dbl)  [unwired: 3 in, 1 out]
      n99 = Fract/Exp String To Number(string=w1023) -> (number=w1027:dbl)  [unwired: 3 in, 1 out]
      n100 = Fract/Exp String To Number(string=w1022) -> (number=w1026:dbl)  [unwired: 3 in, 1 out]
      n101 = Bundle By Name(cluster=T1 {"Barometric Pressure (inches of mercury)"=0.0, "Barometric Pressure (bars)"=0.0, "Air temperature (degC)"=0.0, "Relative humidity (%)"=0.0, "Wind direction, True (deg)"=0.0, "Wind direction, Magnetic (deg)"=0.0, "Wind speed (knots)"=0.0, "Wind speed (m/s)"=0.0} ("Meteorological Data"), "Barometric Pressure (inches of mercury)"=w1029, "Barometric Pressure (bars)"=w1028, "Air temperature (degC)"=w1027, "Relative humidity (%)"=w1026) -> (→"Meteorological Data":T1)
    }
    frame "WIMWV" {
      # "<1> Wind angle, 0.0 to 359.9 degrees, in relation to the vessel’s\nbow/centerline, to the nearest 0.1 degree. If the data for this field is not\nvalid, the field will be blank.\n<2> Reference:\nR = Relative (apparent wind, as felt when standing on the\nmoving ship)\nT = Theoretical (calculated actual wind, as though the vessel\nwere stationary)\n<3> Wind speed, to the nearest tenth of a unit. If the data for this field is\nnot valid, the field will be blank.\n<4> Wind speed units:\nK = km/hr\nM = m/s\nN = knots\nS = statute miles/hr\nIn the PB200 WeatherStation, this field always contains \"N\" (knots).\n<5> Status:\nA = data valid; V = data invalid"
      n102 = call "1A Helper - Generate RegEx.vi"("# Datums"=5) -> ("RegEx"=w1174:string)
      n103 = xnode "Match Regular Expression"("input string"=w1171, "regular expression"=w1174) -> ("submatch 1"=w1173:string, "submatch 2"=w1163:string, "submatch 3"=w1168:string, "submatch 5"=w1167:string)  [unwired: 4 in, 6 out]
      n104 = Fract/Exp String To Number(string=w1173) -> (number=w1164:dbl)  [unwired: 3 in, 1 out]
      n105 = Fract/Exp String To Number(string=w1168) -> (number=w1165:dbl)  [unwired: 3 in, 1 out]
      n106 = Equal?(x=w1167, y="A") -> (x = y?=w1166:bool)
      n107 = case shown="True" w1166 {
        tunnel: w1165 -> [_ w1178]
        tunnel: w1164 -> [_ w1181]
        tunnel: w1163 -> [_ w1180]
        tunnel: w1162 -> [_ w1176]
        frame False {
        }
        frame True {
          # "Convert Ang/Mag to vector & populate globals"
          n108 = Multiply "knots -> m/s"(x=w1178, y=0.51444) -> (x*y=w1179:dbl)
          n109 = case shown="\"T\"" w1180 {
            tunnel: w1179 -> [_ w1184 w1205]
            tunnel: w1181 -> [_ w1189 w1206]
            tunnel: w1176 -> [_ w1186 w1204]
            frame "", Default {
            }
            frame "T" {
              # "Theoretical wind (absolute)"
              n110 = global read "2 Global.vi" "Robot\nHeading"() -> (w1190:T13)
              n111 = Add "Get relative to compass, not boat"(x=w1190, y=w1189) -> (x+y=w1188:T13)
              n112 = call "Velocity Converter- magnitude-heading  to dx-dy.vi"("Magnitude"=w1184, "Heading"=w1188) -> ("Vector Out"=w1195:T14)  [unwired: 9 in]
              n113 = Unbundle By Name(w1195) -> ("North"=w1193:dbl, "East"=w1192:dbl)
              n114 = Quotient & Remainder(x=w1188, y=T13 360.0) -> (x-y*floor(x/y)=w1183:T13)  [unwired: 1 out]
              n115 = Bundle By Name(cluster=T14 {"East"=0.0, "North"=0.0} ("Absolute Wind"), "North"=w1193, "East"=w1192) -> (w1194:T14)
              n116 = case shown="True" w1186 {
                tunnel: [w1196 w1203] -> w1185
                tunnel: w1184 -> [w1196 w1202]
                tunnel: w1183 -> [w1197 w1201]
                tunnel: [w1197 w1200] -> w1182
                frame False {
                }
                frame True {
                  n117 = call "1A Steven's Defilter.vi"("Angle?(F)"=FALSE, "Value In"=w1202) -> ("Filtered Value Out"=w1203:dbl)  [unwired: 3 in]
                  n118 = call "1A Steven's Defilter.vi"("Angle?(F)"=TRUE, "Value In"=w1201) -> ("Filtered Value Out"=w1200:dbl)  [unwired: 3 in]
                }
              }
              n119 = global write "2 Global.vi" "Absolute Wind"(w1194) -> ()
              n120 = global write "2 Global.vi" "Absolute Wind\nDirection (º)"(w1182) -> ()
              n121 = global write "2 Global.vi" "Absolute Wind\nSpeed"(w1185) -> ()
            }
            frame "R" {
              # "Relative wind (apparent)"
              n122 = call "Velocity Converter- magnitude-heading  to dx-dy.vi"("Magnitude"=w1205, "Heading"=w1206) -> ("Vector Out"=w1209:T14)  [unwired: 9 in]
              n123 = case shown="True" w1204 {
                tunnel: [w1214 w1219] -> w1208
                tunnel: [w1215 w1218] -> w1207
                tunnel: w1206 -> [w1215 w1217]
                tunnel: w1205 -> [w1214 w1216]
                frame False {
                }
                frame True {
                  n124 = call "1A Steven's Defilter.vi"("Angle?(F)"=TRUE, "Value In"=w1217) -> ("Filtered Value Out"=w1218:dbl)  [unwired: 3 in]
                  n125 = call "1A Steven's Defilter.vi"("Angle?(F)"=FALSE, "Value In"=w1216) -> ("Filtered Value Out"=w1219:dbl)  [unwired: 3 in]
                }
              }
              n126 = Unbundle By Name(w1209) -> ("North"=w1212:dbl, "East"=w1213:dbl)
              n127 = Bundle By Name(cluster=T15 {"Toward Fore"=0.0, "Toward Starboard"=0.0} ("Apparent Wind"), "Toward Fore"=w1212, "Toward Starboard"=w1213) -> (w1211:T15)
              n128 = global write "2 Global.vi" "Apparent Wind"(w1211) -> ()
              n129 = global write "2 Global.vi" "Apparent Wind\nDirection (º)"(w1207) -> ()
              n130 = global write "2 Global.vi" "Apparent Wind\nSpeed"(w1208) -> ()
            }
          }
        }
      }
      n131 = Bundle By Name(cluster=T10 {"Angle relative to boat (deg)"=0.0, "Wind Data Valid?"=TRUE, "Wind speed (knots)"=0.0, "True (T) or Relative (R)"=""} ("Wind (MWV) Data 2"), "Angle relative to boat (deg)"=w1164, "True (T) or Relative (R)"=w1163, "Wind speed (knots)"=w1165, "Wind Data Valid?"=w1166) -> (→"Wind (MWV) Data":T10)
    }
    frame "WIMWR" {
    }
    frame "WIMWT" {
    }
    frame "YXXDR" {
      n132 = String Subset(string=w1339, length (rest)=1 ("length (rest)")) -> (substring=w1340:string)  [unwired: 1 in]
      n133 = case shown="\"\", Default" w1340 {
        tunnel: w1339 -> [_ w1342 w1481]
        frame "", Default {
        }
        frame "A" {
          # "TYPE B:\n<1> A = angular displacement\n<2> Pitch: oscillation of vessel about its latitudinal axis. Bow moving up is positive. Value reported to the nearest 0.1 degree.\n<3> D = degrees\n<4> PTCH (ID indicating pitch of vessel)\n<5> A = angular displacement\n<6> Roll: oscillation of vessel about its longitudinal axis. Roll to the starboard is positive. Value reported to the nearest 0.1 degree.\n<7> D = degrees\n<8> ROLL (ID indicating roll of vessel)\n<9> Not used\n<10> Not used\n<11> Not used\n<12> Not used\n<13> Not used\n<14> Not used\n<15> Not used\n<16> Not used"
          n134 = call "1A Helper - Generate RegEx.vi"("# Datums"=8) -> ("RegEx"=w1346:string)
          n135 = xnode "Match Regular Expression"("input string"=w1342, "regular expression"=w1346) -> ("submatch 2"=w1344:string, "submatch 6"=w1343:string)  [unwired: 4 in, 19 out]
          n136 = Fract/Exp String To Number(string=w1344) -> (number=w1348:dbl)  [unwired: 3 in, 1 out]
          n137 = Fract/Exp String To Number(string=w1343) -> (number=w1347:dbl)  [unwired: 3 in, 1 out]
          n138 = Bundle By Name(cluster=cluster{"Pitch (deg)":dbl, "Roll (deg)":dbl} {"Pitch (deg)"=103.0, "Roll (deg)"=103.0} ("Transducer (XDR) B Data 2"), "Pitch (deg)"=w1348, "Roll (deg)"=w1347) -> (→"Transducer (XDR) B Data":cluster{"Pitch (deg)":dbl, "Roll (deg)":dbl})
          n139 = Bundle By Name(cluster=T16 {"Pitch"=0.0, "Roll"=0.0} ("Robot Pitch/Roll"), "Pitch"=w1348, "Roll"=w1347) -> (w1349:T16)
          n140 = global write "2 Global.vi" "Robot Pitch/Roll"(w1349) -> ()
        }
        frame "C" {
          # "TYPE A:\n<1> C = temperature\n<2> Calculated “relative” wind chill temperature, degrees Celsius, to the nearest 0.1 degree\n<3> C = degrees C\n<4> WCHR (ID indicating relative wind chill)\n<5> C = temperature\n<6> Calculated “theoretical” wind chill temperature, degrees Celsius, to the nearest 0.1 degree\n<7> C = degrees C\n<8> WCHT (ID indicating theoretical wind chill)\n<9> C = temperature\n<10> Calculated heat index, degrees Celsius, to the nearest 0.1 degree (this field left blank by WeatherStation)\n<11> C = degrees C\n<12> HINX (ID indicating heat index)\n<13> P = pressure\n<14> Actual measured barometric pressure, or \"station pressure\", bars, to the nearest 0.001 bar\n<15> B = bars\n<16> STNP (ID indicating station pressure)"
          n141 = call "1A Helper - Generate RegEx.vi"("# Datums"=16) -> ("RegEx"=w1487:string)
          n142 = xnode "Match Regular Expression"("input string"=w1481, "regular expression"=w1487) -> ("submatch 2"=w1485:string, "submatch 6"=w1484:string, "submatch 10"=w1483:string, "submatch 14"=w1482:string)  [unwired: 4 in, 17 out]
          n143 = Fract/Exp String To Number(string=w1485) -> (number=w1491:dbl)  [unwired: 3 in, 1 out]
          n144 = Fract/Exp String To Number(string=w1484) -> (number=w1490:dbl)  [unwired: 3 in, 1 out]
          n145 = Fract/Exp String To Number(string=w1483) -> (number=w1489:dbl)  [unwired: 3 in, 1 out]
          n146 = Fract/Exp String To Number(string=w1482) -> (number=w1488:dbl)  [unwired: 3 in, 1 out]
          n147 = Bundle By Name(cluster=T11 {"Calc. Relative Wind Chill (degC)"=0.0, "Calc. Theoretical Wind Chill (degC)"=0.0, "Calc. Heat Index (degC)"=0.0, "Meas. Barometric Pressure (bars)"=0.0} ("Transducer (XDR) A Data 2"), "Calc. Relative Wind Chill (degC)"=w1491, "Calc. Theoretical Wind Chill (degC)"=w1490, "Calc. Heat Index (degC)"=w1489, "Meas. Barometric Pressure (bars)"=w1488) -> (→"Transducer (XDR) A Data":T11)
        }
      }
    }
  }
